vi "CoreTestHarness.vi"() -> ()   [LabVIEW 2017]
uses:
  <vilib>/NI/PowerElectronicsControl/SVPWM/SVPWM/SwitchPositions.ctl
  AFE/Outputs.ctl
  AFE/Inputs.ctl
  <vilib>/Platform/TimedLoop/XDataNode/timing_clust.ctl
  <vilib>/Platform/TimedLoop/XDataNode/nitl_modes.ctl
  <vilib>/Platform/TimedLoop/XDataNode/wakeup.ctl
  <instrlib>/_niInstr/Instruction Framework/v1/FPGA/Helper Classes/Single Address Space Collection/Single Address Space Collection.lvclass
  C:/Program Files (x86)/National Instruments/LabVIEW 2017/instr.lib/_niInstr/Instruction Framework/v1/FPGA/Interfaces/Address Space Collection/Address Space Collection.lvclass
  <instrlib>/_niInstr/FIFO Register Bus/v1/FPGA/niInstr FIFO Register Bus v1 FPGA.lvclass
  C:/Program Files (x86)/National Instruments/LabVIEW 2017/instr.lib/_niInstr/Instruction Framework/v1/FPGA/Interfaces/Instruction Producer/Instruction Producer.lvclass
  <vilib>/rvi/Emulation/niFpgaGetClockAttributes.vi
  <vilib>/rvi/Emulation/niFpgaSctlEmulationGetInTimedLoop.vi
  <vilib>/rvi/Emulation/niFpgaEmulationReportErrorSimple.vi
  <vilib>/rvi/eio/common/nirviEmuTemplateMethod_errors.vi
  <vilib>/rvi/Emulation/niFpgaCriticalErrorInLSC.vi
  <vilib>/rvi/Emulation/niFpgaProcessEmulError.vi
  <vilib>/rvi/DataTransferAndStorage/Container/Common/niFpgaContainerExecOnDevCompGetState.vi
  <vilib>/rvi/Emulation/niFpgaEmulationIsFPGAContextNoSignature.vi
  <vilib>/rvi/DataTransferAndStorage/Container/Common/niFpgaContainerGetUniqueNameForEmu.vi
  <vilib>/rvi/Memory/Memory_Emulation/niFpgaMemoryEmulationCacheClearOnFirstRun.vi
  <vilib>/rvi/Memory/Memory_Emulation/nirvimemoryEmulationManagerCache_MakeExclusive.vi
  <vilib>/rvi/Memory/Memory_Emulation/niFpgaMemoryEmulationValidateCache.vi
  <vilib>/rvi/Memory/Memory_Emulation/nirvimemoryEmulationManagerCache_InsertValue.vi
  <vilib>/Utility/error.llb/Clear Errors.vi
  <vilib>/rvi/Memory/Memory_Emulation/nirvimemoryEmulationManagerCache_ReleaseExclusive.vi
  <vilib>/rvi/Memory/Memory_Emulation/nirvimemoryEmulationManagerCache_GetValue.vi
  <vilib>/rvi/Memory/Memory_Emulation/nirvimemoryEmulationManagerCache_SetValue.vi
  <userlib>/_NI FLP Library/addons/PowerElectronics/SpaceVectorPWM/FlpLib SpaceVectorPWM 0.vi
  <vilib>/Platform/TimedLoop/XDataNode/XDataNode.xnode
  <vilib>/eio/EIONode/EIONode.xnode
  <vilib>/rvi/DataTransferAndStorage/Container/XNode/niFpgaContainer.xnode
  <vilib>/rvi/DataTransferAndStorage/Register/Emulation/niFpgaRegisterEmulationRefIn.vi
  <vilib>/Platform/TimedLoop/XDataNode/XDNodeRunTimeDep.lvlib
  <instrlib>/_niInstr/Instruction Framework/v1/FPGA/Top Level Bus/Register Configuration/Register Configuration.lvclass
  <vilib>/NI/PowerElectronicsControl/ScaleAndLimit/Core/ScaleAndLimit.lvlib
  <vilib>/NI/PowerElectronicsControl/ScaleAndLimit/Core/AddressSpace.lvclass
  <vilib>/NI/PowerElectronicsControl/WaveformAcq/FPGA/WaveformAddressSpace.lvclass
  <vilib>/NI/PowerElectronicsControl/SVPWM/SVPWM/SVPWM.lvlib
  <vilib>/NI/PowerElectronicsControl/SVPWM/SVPWM/AddressSpace.lvclass
  AFE/ActiveFrontEnd.lvlib
  AFE/AddressSpace.lvclass
panel:
  in  "Inputs":T1
  out "Outputs":T2
  out "SwitchPositions":T3
  in  "enable":bool
  in  "engauge":bool
  out "Deadtime":u8
  out "Period":u32
  in  "fifo reg bus ctrl 0":u32
  out "fifo reg bus status 0":u32
  out "fifo reg bus data 0":u64
  out "scaled":sgl[](array[numeric])
  out "relativeTimestamp":i32
  out "SimultaneousAILoopRate":u32
  out "LimitsFlag":bool
  out "Iw_B":sgl
  out "Iv_B":sgl
  out "Iu_B":sgl
  out "Vw_B":sgl
  out "Vv_B":sgl
  out "Vu_B":sgl
  out "VDC_LinkB":sgl
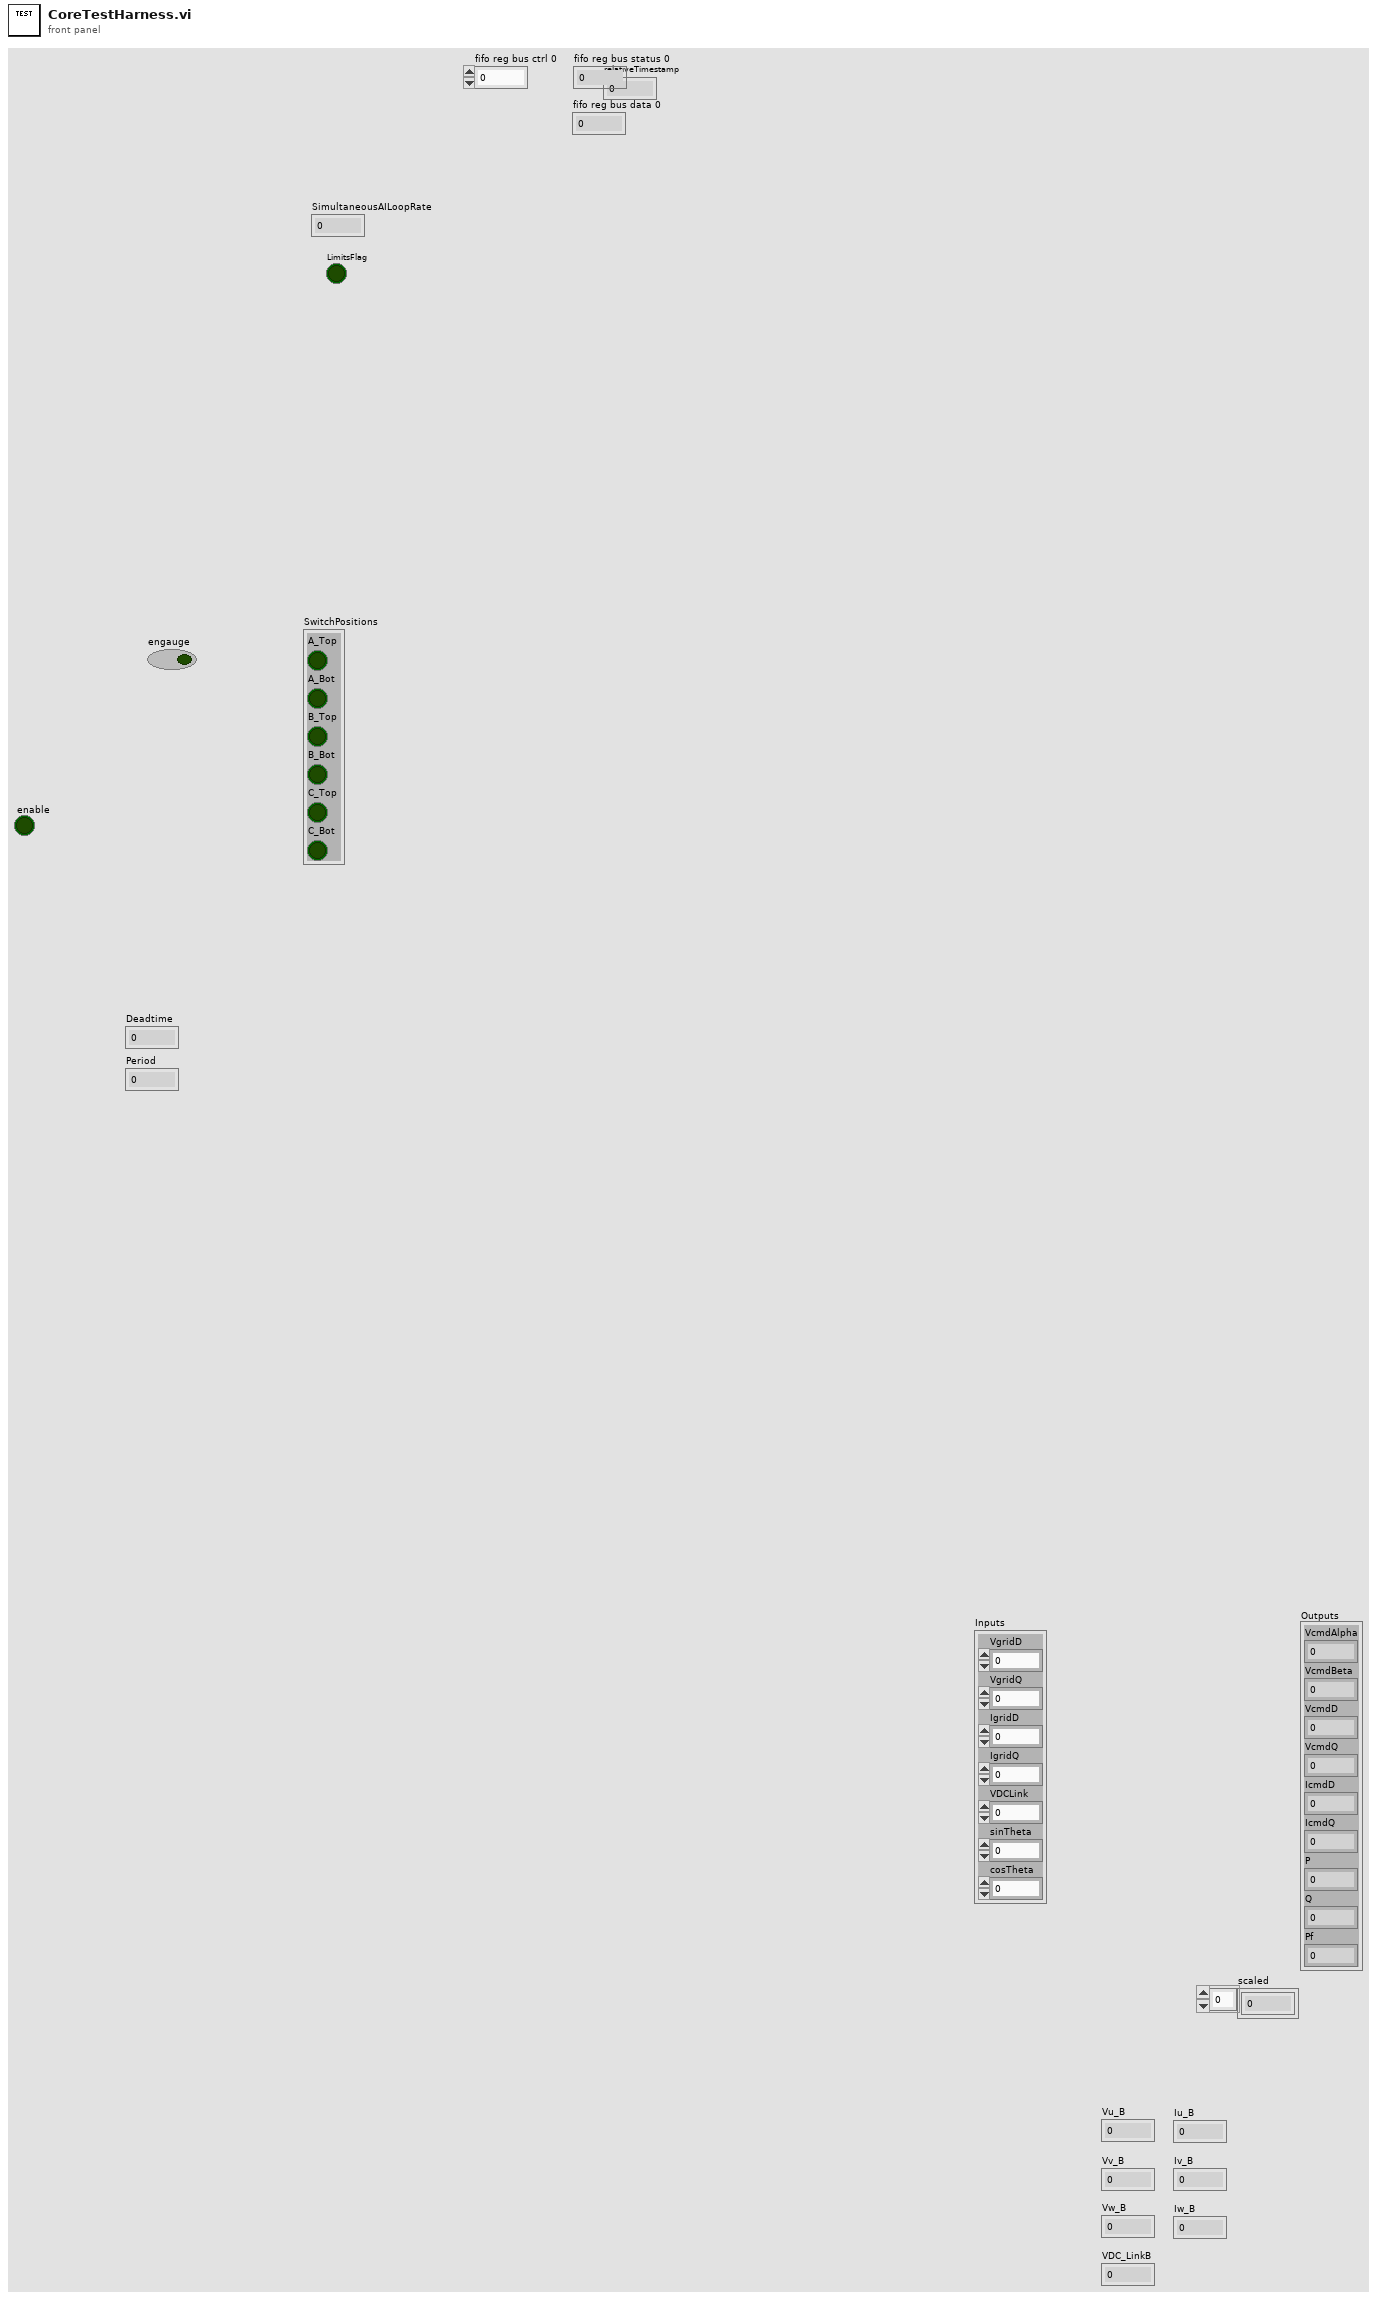
[diagram p1: front panel]
types:
  T1 = typedef "ActiveFrontEnd.lvlib/Inputs.ctl" = cluster{"VgridD":sgl, "VgridQ":sgl, "IgridD":sgl, "IgridQ":sgl, "VDCLink":sgl, "sinTheta":sgl, "cosTheta":sgl}
  T2 = typedef "ActiveFrontEnd.lvlib/Outputs.ctl" = cluster{"VcmdAlpha":sgl, "VcmdBeta":sgl, "VcmdD":sgl, "VcmdQ":sgl, "IcmdD":sgl, "IcmdQ":sgl, "P":sgl, "Q":sgl, "Pf":sgl}
  T3 = typedef "SVPWM.lvlib/SwitchPositions.ctl" = cluster{"A_Top":bool, "A_Bot":bool, "B_Top":bool, "B_Bot":bool, "C_Top":bool, "C_Bot":bool}
  T4 = typedef "XDNodeRunTimeDep.lvlib/timing_clust.ctl" = cluster{"Expected End [f-1]":u64, "Actual End [f-1]":u64, "Finished Late? [f-1]":bool, "Expected End [i-1]":u64, "Actual End [i-1]":u64, "Finished Late? [i-1]":bool, "Expected Start [i]":u64, "Actual Start [i]":u64, "Expected Start [f]":u64, "Actual Start [f]":u64, "Source Name":string, "Structure Name":string, "Period":i64, "Deadline":i64, "Offset":i64, "Start":i64, "Priority":i32, "Timeout":i32, "Mode":T5, "Wakeup Reason":T6, "Error":errorcluster, "Source Type":string, "Secondary Source Type":string, "Global End Time":u64, "Global Start Time":u64, "Frame Duration":u64, "Iteration Duration":u64, "Assigned CPU":i32, "I/O Scan Engine Mode":u32}
  T5 = typedef "XDNodeRunTimeDep.lvlib/nitl_modes.ctl" = enum32{"No Change", "Process missed periods, maintain original phase", "Discard missed periods, maintain original phase", "Process missed periods, ignore original phase", "Discard missed periods, ignore original phase"}
  T6 = typedef "XDNodeRunTimeDep.lvlib/wakeup.ctl" = enum32{"Normal", "Aborted", "Asynchronous wakeup", "Timing source error", "Timed loop error", "Timeout"}
  T7 = typedef "SVPWM.lvlib/Parameters.ctl" = cluster{"Deadtime":refnum<k21>, "Period":refnum<k21>, "A_timing":refnum<k21>, "B_timing":refnum<k21>, "C_timing":refnum<k21>}
  T8 = typedef "ActiveFrontEnd.lvlib/ControllerRegisters.ctl" = cluster{"Parameters":refnum<k21>, "VDCLinkToP_PISettings":refnum<k21>, "ID_to_VD_PISettings":refnum<k21>, "IQ_to_VQ_PISettings":refnum<k21>}
  T9 = typedef "ON_OFF.ctl" = cluster{"ON":u32, "OFF":u32}
  T10 = typedef "ScaleAndLimit.lvlib/LimitsRegisters.ctl" = cluster{"HighLimits":refnum<k21>, "LowLimits":refnum<k21>, "ClearLimits":refnum<k21>, "LimitsFlag":refnum<k21>}
  T11 = typedef "ScaleAndLimit.lvlib/ConfigRegisters.ctl" = cluster{"LimitsEnabled":refnum<k21>, "UnscaledHighLimit":refnum<k21>, "UnscaledLowLimit":refnum<k21>, "B":refnum<k21>, "M":refnum<k21>}
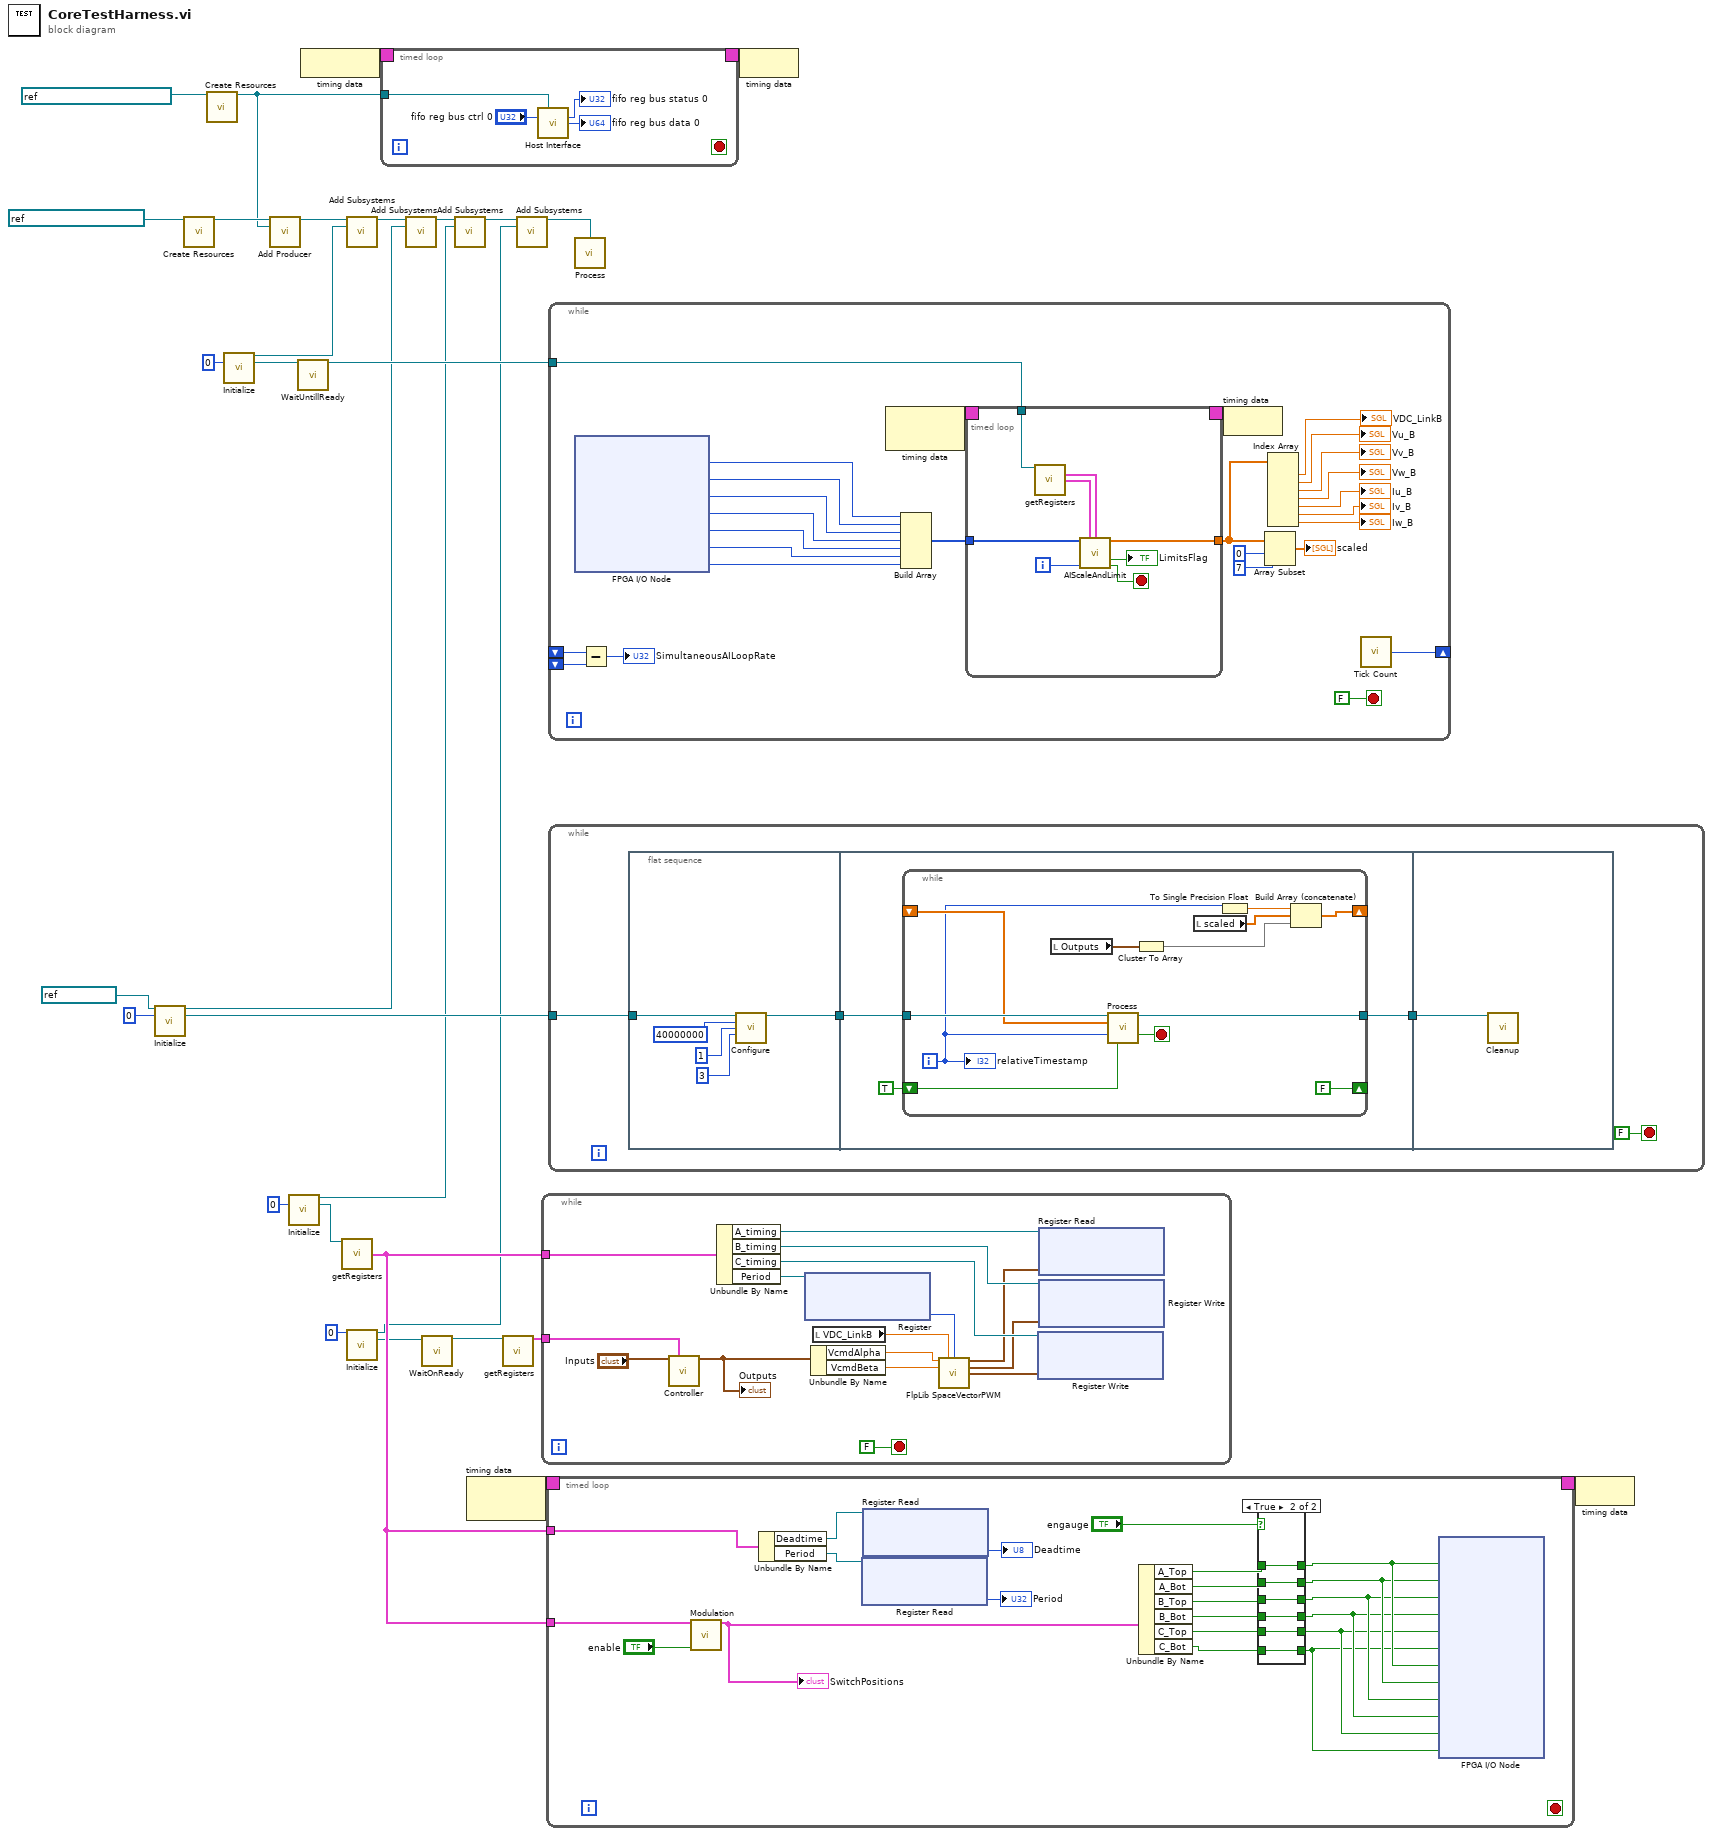
[diagram p0: block diagram]
diagram:
  n1 = call <vilib>:"Initialize.vi"("DMA FIFO"=refnum<k21> "DataSGL0" ("FIFO Out"), "instance"=u8 0) -> ("subsystem"=w21:refnum<class "Single Address Space Collection.lvclass">, "AddressSpace"=w23:refnum<class "WaveformAddressSpace.lvclass">)  [unwired: 12 in]
  n2 = call <instrlib>:"Create Resources.vi"("register clock"=refnum<k21> "40 MHz Onboard Clock") -> ("register configuration"=w17:refnum<class "Register Configuration.lvclass">)  [unwired: 14 in]
  n3 = call <instrlib>:"Create Resources.vi"("instruction fifo"=refnum<k21> "reg.host instruction fifo 0") -> ("fifo register bus"=w15:refnum<class "niInstr FIFO Register Bus v1 FPGA.lvclass">)  [unwired: 14 in]
  n4 = call <vilib>:"Initialize.vi"("instance"=u8 0) -> ("subsystem"=w29:refnum<class "Single Address Space Collection.lvclass">, "AddressSpace"=w27:refnum<class "AddressSpace.lvclass">)  [unwired: 13 in]
  n5 = call <instrlib>:"Add Producer.vi"("register configuration in"=w17, "instruction producer"=w15) -> ("register configuration out"=w16:refnum<class "Register Configuration.lvclass">)  [unwired: 13 in]
  n6 = call <vilib>:"Initialize.vi"("instance"=u8 0) -> ("subsystem"=w8:refnum<class "Single Address Space Collection.lvclass">, "AddressSpace"=w11:refnum<class "AddressSpace.lvclass">)  [unwired: 13 in]
  n7 = call <vilib>:"WaitUntillReady.vi"("AddressSpace in"=w27) -> ("AddressSpace out"=w26:refnum<class "AddressSpace.lvclass">)  [unwired: 14 in]
  n8 = node-c288() -> (w20:T4)
  n9 = call <vilib>:"getRegisters.vi"("AddressSpace in"=w11) -> ("Parameters"=w10:T7)  [unwired: 13 in, 1 out]
  n10 = call <instrlib>:"Add Subsystems.vi"("register configuration in"=w16, "subsystems"=w29) -> ("register configuration out"=w22:refnum<class "Register Configuration.lvclass">)  [unwired: 13 in]
  n11 = call <vilib>:"Initialize.vi"("instance"=u8 0) -> ("subsysytem"=w3:refnum<class "Single Address Space Collection.lvclass">, "AddressSpace"=w6:refnum<class "AddressSpace.lvclass">)  [unwired: 13 in]
  n12 = timed-loop {
    timing: w20 -> [_]
    timing-out: [_] -> w19
    tunnel: w15 -> [w34]
    stop <- _ stop-if-true
    n13 = call <instrlib>:"Host Interface.vi"("fifo register bus"=w34, "fifo reg bus ctrl 0"="fifo reg bus ctrl 0") -> ("fifo reg bus status 0"=→"fifo reg bus status 0":u32, "fifo reg bus data 0"=→"fifo reg bus data 0":u64)  [unwired: 12 in]
  }
  n14 = call <instrlib>:"Add Subsystems.vi"("register configuration in"=w22, "subsystems"=w21) -> ("register configuration out"=w9:refnum<class "Register Configuration.lvclass">)  [unwired: 13 in]
  n15 = call "WaitOnReady.vi"("AddressSpace in"=w6) -> ("AddressSpace out"=w5:refnum<class "AddressSpace.lvclass">)  [unwired: 14 in]
  n16 = call <instrlib>:"Add Subsystems.vi"("register configuration in"=w9, "subsystems"=w8) -> ("register configuration out"=w2:refnum<class "Register Configuration.lvclass">)  [unwired: 13 in]
  n17 = node-c288() -> (w14:T4)  [unwired: 1 in]
  n18 = call <vilib>:"getRegisters.vi"("AddressSpace in"=w5) -> ("CntlRegisters"=w4:T8)  [unwired: 14 in]
  n19 = call <instrlib>:"Add Subsystems.vi"("register configuration in"=w2, "subsystems"=w3) -> ("register configuration out"=w1:refnum<class "Register Configuration.lvclass">)  [unwired: 13 in]
  n20 = while {
    tunnel: w10 -> [w38]
    tunnel: w4 -> [w37]
    stop <- FALSE stop-if-true
    n21 = call "Controller.vi"("Inputs"="Inputs", "Registers"=w37) -> ("Outputs"=w39:T2)  [unwired: 13 in]
    "Outputs" <- w39
    n22 = Unbundle By Name(w38) -> ("A_timing"=w47:refnum<k21>, "B_timing"=w46:refnum<k21>, "C_timing"=w45:refnum<k21>, "Period"=w49:refnum<k21>)
    n23 = xnode "Register"("Register In"=w49) -> ("Data"=w48:u32)  [unwired: 1 out]
    n24 = Unbundle By Name(w39) -> ("VcmdAlpha"=w51:sgl, "VcmdBeta"=w50:sgl)
    n25 = local read "VDC_LinkB"() -> (w41:sgl)
    n26 = call-poly <userlib>:"FlpLib SpaceVectorPWM.vi"("ref_alpha"=w51, "ref_max"=w41, "Period"=w48, "ref_beta"=w50) -> ("A"=w44:T9, "B"=w43:T9, "C"=w42:T9)  [unwired: 8 in, 1 out]
    n27 = xnode "Register Write"("Data"=w42, "Register In"=w45) -> ()  [unwired: 1 out]
    n28 = xnode "Register Read"("Data"=w44, "Register In"=w47) -> ()  [unwired: 1 out]
    n29 = xnode "Register Write"("Data"=w43, "Register In"=w46) -> ()  [unwired: 1 out]
  }
  n30 = timed-loop {
    timing: w14 -> [_]
    timing-out: [_] -> w13
    tunnel: w10 -> [w68]
    tunnel: w10 -> [w53]
    stop <- _ stop-if-true
    n31 = call <vilib>:"Modulation.vi"("Parameters"=w53, "enable"="enable") -> ("SwitchPositions"=w66:T3)  [unwired: 13 in]
    "SwitchPositions" <- w66
    n32 = Unbundle By Name(w68) -> ("Deadtime"=w72:refnum<k21>, "Period"=w71:refnum<k21>)
    n33 = xnode "Register Read"("Register In"=w71) -> ("Data"=→"Period":u32)  [unwired: 1 out]
    n34 = xnode "Register Read"("Register In"=w72) -> ("Data"=→"Deadtime":u8)  [unwired: 1 out]
    n35 = Unbundle By Name(w66) -> ("A_Top"=w65:bool, "A_Bot"=w64:bool, "B_Top"=w63:bool, "B_Bot"=w62:bool, "C_Top"=w61:bool, "C_Bot"=w60:bool)
    n36 = case shown="True" "engauge" {
      tunnel: w65 -> [_ w79]
      tunnel: [_ w79] -> w59
      tunnel: w64 -> [_ w78]
      tunnel: [_ w78] -> w58
      tunnel: w63 -> [_ w77]
      tunnel: [_ w77] -> w57
      tunnel: w62 -> [_ w76]
      tunnel: [_ w76] -> w56
      tunnel: w61 -> [_ w75]
      tunnel: [_ w75] -> w55
      tunnel: w60 -> [_ w74]
      tunnel: [_ w74] -> w54
      frame False {
      }
      frame True {
      }
    }
    n37 = xnode "FPGA I/O Node"("s2B / uTOPB"=w59, "s1B / uBOTB"=w58, "s4B / vTOPB"=w57, "s3B  / vBOTB"=w56, "s6B / wTOPB"=w55, "s5B / wBOTB"=w54, "HB1B-TOP"=w59, "HB1B-BOT"=w58, "HB2B-TOP"=w57, "HB2B-BOT"=w56, "HB3B-TOP"=w55, "HB3B-BOT"=w54) -> ()  [unwired: 12 in, 12 out]
  }
  n38 = while {
    shift-right: [w107] -> _
    shift-left: _ -> [w106]
    shift-left: _ -> [w105]
    tunnel: w26 -> [w101]
    stop <- FALSE stop-if-true
    n39 = xnode "FPGA I/O Node"() -> ("AI4+ / VDC_Link_B"=w99:i16, "AI5+ / Vu_B"=w98:i16, "AI6+ / Vv_B"=w97:i16, "AI7+ / Vw_B"=w96:i16, "AI0+ / Iu_B"=w95:i16, "AI1+ / Iv_B"=w94:i16, "AI2+ / Iw_B"=w93:i16)  [unwired: 7 in, 7 out]
    n40 = Subtract(x=w106, y=w105) -> (x-y=→"SimultaneousAILoopRate":u32)
    n41 = node-c288() -> (w103:T4)  [unwired: 1 in]
    n42 = Build Array(w99, w98, w97, w96, w95, w94, w93) -> (w100:i16[])
    n43 = timed-loop {
      timing: w103 -> [_]
      timing-out: [_] -> w102
      tunnel: w100 -> [w116]
      tunnel: [w115] -> w85
      tunnel: w101 -> [w113]
      i -> [w110]
      stop <- w114 stop-if-true
      n44 = call <vilib>:"getRegisters.vi"("AddressSpace in"=w113) -> ("LimitsRegisters"=w111:T10, "ConfigRegisters"=w112:T11)  [unwired: 12 in, 1 out]
      n45 = call <vilib>:"AIScaleAndLimit.vi"("UnscaledAI"=w116, "ConfigRegisters"=w112, "LimitsRegisters"=w111, "index"=w110) -> ("ScaledAI"=w115:sgl[], "Limited"=→"LimitsFlag":bool, "output valid"=w114:bool)  [unwired: 9 in]
    }
    n46 = node-c288(w102) -> ()
    n47 = Array Subset(array=w85, index=0, length=7) -> (→"scaled":sgl[])
    n48 = Index Array(array=w85) -> (element #1=→"VDC_LinkB":sgl, element #2=→"Vu_B":sgl, element #3=→"Vv_B":sgl, element #4=→"Vw_B":sgl, element #5=→"Iu_B":sgl, element #6=→"Iv_B":sgl, element #7=→"Iw_B":sgl)  [unwired: 7 in]
    n49 = call "Tick Count"() -> ("Tick Count(Ticks)"=w107:u32)
  }
  n50 = while {
    tunnel: w23 -> [w121]
    stop <- FALSE stop-if-true
    n51 = flat-sequence {
      tunnel: [w125] -> w123
      tunnel: w121 -> [w126]
      tunnel: w123 -> [w132]
      tunnel: [w131] -> w122
      tunnel: w122 -> [w145]
      frame #0 {
        n52 = call <vilib>:"Configure.vi"("WaveformAddressSpace in"=w126, "oclk_freq"=u32 40000000, "oclk_mult"=u32 1, "UnderflowMargin"=u32 3 ("y")) -> ("WaveformAddressSpace out"=w125:refnum<class "WaveformAddressSpace.lvclass">)  [unwired: 11 in]
      }
      frame #1 {
        n53 = while {
          shift-right: [w143] -> _
          shift-left: _ -> [w138]
          shift-right: [FALSE] -> _
          shift-left: TRUE -> [w139]
          tunnel: w132 -> [w141]
          tunnel: [w140] -> w131
          i -> [w137]
          stop <- w142 stop-if-true
          n54 = local read "Outputs"() -> (w134:T2)
          n55 = call <instrlib>:"Process.vi"("WaveformAddressSpace in"=w141, "Data"=w138, "Iteration"=w137, "FirstIteration"=w139) -> ("WaveformAddressSpace out"=w140:refnum<class "WaveformAddressSpace.lvclass">, "stop"=w142:bool)  [unwired: 8 in, 2 out]
          n56 = Cluster To Array(cluster=w134) -> (array=w133:sgl[])
          n57 = local read "scaled"() -> (w135:sgl[])
          n58 = To Single Precision Float(number=w137) -> (single precision float=w136:sgl)
          n59 = Build Array (concatenate)(w136, w135, w133) -> (w143:sgl[])
          "relativeTimestamp" <- w137
        }
      }
      frame #2 {
        n60 = call <vilib>:"Cleanup.vi"("WaveformAddressSpace in"=w145) -> ()  [unwired: 14 in, 1 out]
      }
    }
  }
  n61 = call <instrlib>:"Process.vi"("register configuration"=w1) -> ()  [unwired: 15 in]
  n62 = node-c288(w19) -> ()
  n63 = node-c288(w13) -> ()
